vi "rethinkdb_example_ui.vi"() -> ()   [LabVIEW 2017]
uses:
  rethinkdb/rethinkdb.lvlib
panel:
  out "generated_keys":string[](array[string])
  in  "insert":bool
  in  "json":string
  in  "launch":bool
  in  "table_drop":bool
  in  "table_create":bool
  in  "table":string="mytable"
  out "table list":string[](array[string])
  in  "table_list":bool
  out "db list":string[](array[string])
  in  "db_list":bool
  in  "db":string="mydb"
  in  "db_drop":bool
  in  "db_create":bool
  out "error":errorcluster
  out "status":string
  in  "disconnect":bool
  out "is_connected?":bool
  in  "connect":bool
  in  "host":string="localhost"
  in  "port":u16=28015
  in  "ms timeout":i32=10000
  in  "user":string="admin"
  in  "password":string
  # "Connection"
  # "Database"
  # "Table"
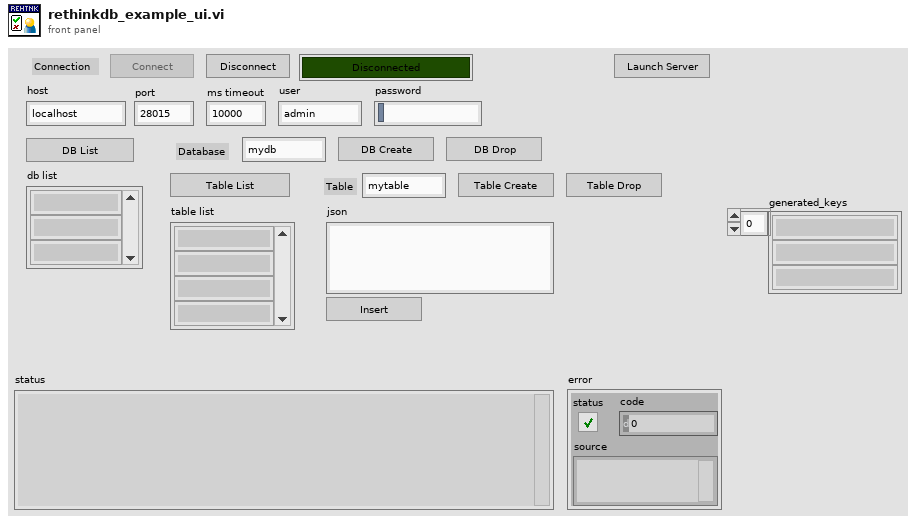
[diagram p1: front panel]
types:
  T1 = typedef "rethinkdb.lvlib/refnum.ctl" = refnum<k1>
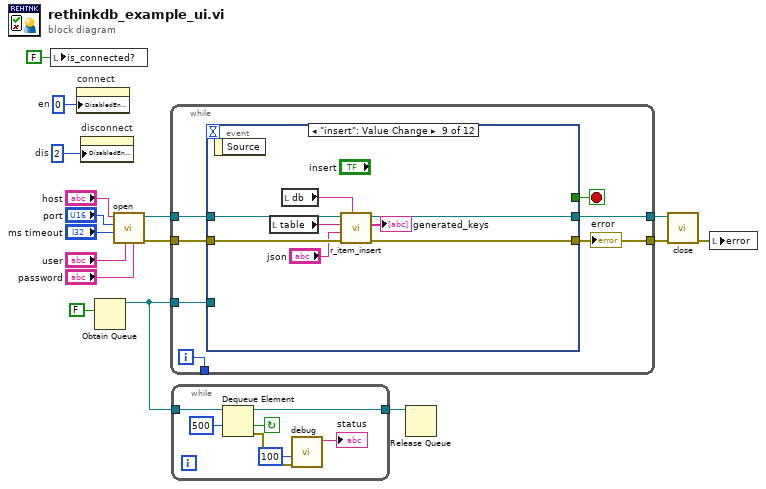
[diagram p0: block diagram]
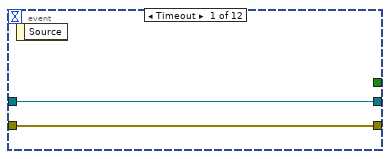
[diagram p2: hidden frame]
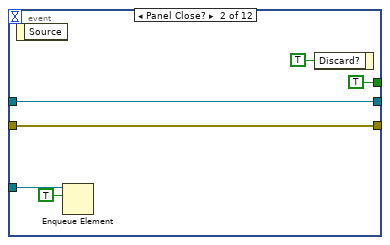
[diagram p3: hidden frame]
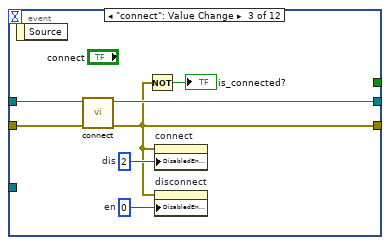
[diagram p4: hidden frame]
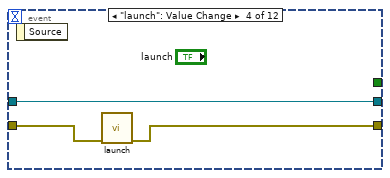
[diagram p5: hidden frame]
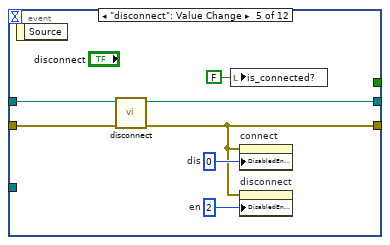
[diagram p6: hidden frame]
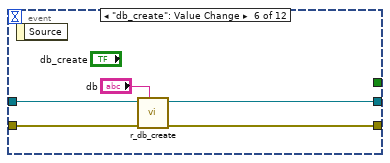
[diagram p7: hidden frame]
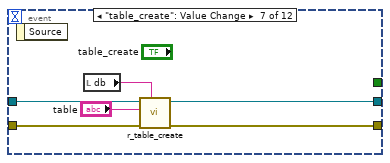
[diagram p8: hidden frame]
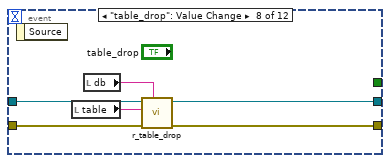
[diagram p9: hidden frame]
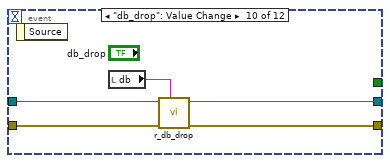
[diagram p10: hidden frame]
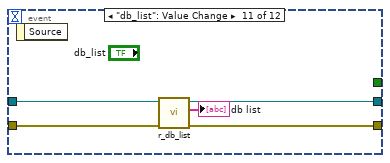
[diagram p11: hidden frame]
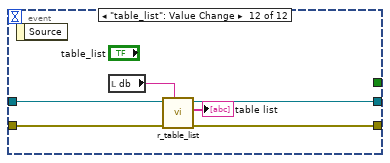
[diagram p12: hidden frame]
diagram:
  w6 = 0  # en
  w7 = u8 2  # dis
  n1 = local write "is_connected?"(FALSE ("is_connected?")) -> ()
  n2 = property on="connect" class="Bool"("DisabledEnum"=w6) -> ()  [unwired: 2 in, 2 out]
  n3 = property on="disconnect" class="Bool"("DisabledEnum"=w7) -> ()  [unwired: 2 in, 2 out]
  n4 = Obtain Queue(element data type=FALSE) -> (queue out=w3:refnum<queue>)  [unwired: 4 in, 2 out]
  n5 = call "open.vi"("password (\"\")"="password", "user (\"admin\")"="user", "ms timeout (10000)"="ms timeout", "port (28015)"="port", "host (\"localhost\")"="host") -> ("error out"=w16:errorcluster, "rethinkdb"=w15:T1)  [unwired: 5 in]
  n6 = while {
    tunnel: w16 -> [w23]
    tunnel: w15 -> [w22]
    tunnel: [w19] -> w13
    tunnel: [w21] -> w14
    tunnel: [w18] -> _
    tunnel: w3 -> [w17]
    i -> [w18]
    stop <- w20 stop-if-true
    n7 = event shown="[8] \"insert\": Value Change" {
      selector: _ -> [_ _ _ _ _ _ _ _ _ _ _ _]
      dyn-events: _ -> [_ _ _ _ _ _ _ _ _ _ _ _]
      timeout: _ -> [_ _ _ _ _ _ _ _ _ _ _ _]
      tunnel: w23 -> [w25 w31 w38 w41 w46 w53 w59 w65 w73 w78 w83 w89]
      tunnel: w22 -> [w24 w30 w37 w39 w45 w51 w58 w64 w71 w76 w82 w88]
      tunnel: [w25 w31 w33 w40 w43 w52 w56 w61 w72 w77 w80 w87] -> w19
      tunnel: [w24 w30 w36 w39 w44 w50 w57 w60 w70 w75 w81 w86] -> w21
      tunnel: [_ TRUE _ _ _ _ _ _ _ _ _ _] -> w20
      tunnel: w17 -> [_ w27 _ _ _ _ _ _ _ _ _ _]
      event Timeout {
        n8 = event-data() -> ()  [unwired: 1 in, 1 out]
      }
      event Panel Close? {
        n9 = event-data() -> ()  [unwired: 1 in, 1 out]
        n10 = Enqueue Element(queue=w27, element=TRUE) -> ()  [unwired: 2 in, 3 out]
        n11 = event-data("Discard?"=TRUE) -> ()  [unwired: 1 in, 1 out]
      }
      event "connect": Value Change {
        w34 = 2  # dis
        w35 = 0  # en
        n12 = event-data() -> ()  [unwired: 1 in, 1 out]
        n13 = call "connect.vi"("error in (no error)"=w38, "rethinkdb in"=w37) -> ("error out"=w33:errorcluster, "rethinkdb out"=w36:T1)  [unwired: 8 in]
        n14 = Not(x=w33) -> (.not. x?=→"is_connected?":bool)
        n15 = property on="connect" class="Bool"(error in=w33, "DisabledEnum"=w34) -> ()  [unwired: 1 in, 2 out]
        n16 = property on="disconnect" class="Bool"(error in=w33, "DisabledEnum"=w35) -> ()  [unwired: 1 in, 2 out]
      }
      event "launch": Value Change {
        n17 = event-data() -> ()  [unwired: 1 in, 1 out]
        n18 = call "launch.vi"("error in (no error)"=w41) -> ("error out"=w40:errorcluster)  [unwired: 10 in]
      }
      event "disconnect": Value Change {
        w47 = 0  # dis
        w48 = 2  # en
        n19 = event-data() -> ()  [unwired: 1 in, 1 out]
        n20 = call "disconnect.vi"("error in (no error)"=w46, "rethinkdb in"=w45) -> ("error out"=w43:errorcluster, "rethinkdb out"=w44:T1)  [unwired: 8 in]
        n21 = local write "is_connected?"(FALSE ("is_connected?")) -> ()
        n22 = property on="connect" class="Bool"(error in=w43, "DisabledEnum"=w47) -> ()  [unwired: 1 in, 2 out]
        n23 = property on="disconnect" class="Bool"(error in=w43, "DisabledEnum"=w48) -> ()  [unwired: 1 in, 2 out]
      }
      event "db_create": Value Change {
        n24 = event-data() -> ()  [unwired: 1 in, 1 out]
        n25 = call "r_db_create.vi"("db"="db", "error in (no error)"=w53, "rethinkdb in"=w51) -> ("error out"=w52:errorcluster, "rethinkdb out"=w50:T1)  [unwired: 5 in, 2 out]
      }
      event "table_create": Value Change {
        n26 = event-data() -> ()  [unwired: 1 in, 1 out]
        n27 = local read "db"() -> (w54:string)
        n28 = call "r_table_create.vi"("db"=w54, "error in (no error)"=w59, "table"="table", "rethinkdb in"=w58) -> ("error out"=w56:errorcluster, "rethinkdb out"=w57:T1)  [unwired: 4 in, 2 out]
      }
      event "table_drop": Value Change {
        n29 = event-data() -> ()  [unwired: 1 in, 1 out]
        n30 = local read "table"() -> (w62:string)
        n31 = local read "db"() -> (w63:string)
        n32 = call "r_table_drop.vi"("db"=w63, "error in (no error)"=w65, "table"=w62, "rethinkdb in"=w64) -> ("error out"=w61:errorcluster, "rethinkdb out"=w60:T1)  [unwired: 4 in, 2 out]
      }
      event "insert": Value Change {
        n33 = event-data() -> ()  [unwired: 1 in, 1 out]
        n34 = local read "table"() -> (w68:string)
        n35 = local read "db"() -> (w69:string)
        n36 = call "r_item_insert.vi"("db"=w69, "error in (no error)"=w73, "json"="json", "table"=w68, "rethinkdb in"=w71) -> ("error out"=w72:errorcluster, "generated_keys"=→"generated_keys":string[], "rethinkdb out"=w70:T1)  [unwired: 3 in, 1 out]
      }
      event "db_drop": Value Change {
        n37 = event-data() -> ()  [unwired: 1 in, 1 out]
        n38 = local read "db"() -> (w74:string)
        n39 = call "r_db_drop.vi"("db"=w74, "error in (no error)"=w78, "rethinkdb in"=w76) -> ("error out"=w77:errorcluster, "rethinkdb out"=w75:T1)  [unwired: 5 in, 2 out]
      }
      event "db_list": Value Change {
        n40 = event-data() -> ()  [unwired: 1 in, 1 out]
        n41 = call "r_db_list.vi"("error in (no error)"=w83, "rethinkdb in"=w82) -> ("error out"=w80:errorcluster, "db list"=→"db list":string[], "rethinkdb out"=w81:T1)  [unwired: 7 in]
      }
      event "table_list": Value Change {
        n42 = event-data() -> ()  [unwired: 1 in, 1 out]
        n43 = local read "db"() -> (w84:string)
        n44 = call "r_table_list.vi"("db"=w84, "error in (no error)"=w89, "rethinkdb in"=w88) -> ("error out"=w87:errorcluster, "table list"=→"table list":string[], "rethinkdb out"=w86:T1)  [unwired: 6 in]
      }
    }
    "error" <- w19
  }
  n45 = while {
    tunnel: w3 -> [w96]
    tunnel: [w93] -> w2
    stop <- w91 continue-if-true
    n46 = Dequeue Element(queue=w96, timeout in ms (-1)=500) -> (queue out=w93:refnum<queue>, timed out?=w91:bool, error out=w95:errorcluster)  [unwired: 1 in, 1 out]
    n47 = call "debug.vi"("error in (no error)"=w95, "ms update rate (1000)"=u32 100) -> ("debug"=→"status":string)  [unwired: 8 in, 1 out]
  }
  n48 = Release Queue(queue=w2) -> ()  [unwired: 2 in, 3 out]
  n49 = call "close.vi"("error in (no error)"=w13, "rethinkdb"=w14) -> ("error out"=w5:errorcluster)  [unwired: 9 in]
  n50 = local write "error"(w5) -> ()
